vi "test Deployment Import Configuration.vi"(8 "error in":errorcluster, 11 "TestCase in":refnum<class "Deployment.lvclass">) -> (0 "error out":errorcluster, 3 "TestCase out":refnum<class "Deployment.lvclass">)   [LabVIEW 2020, in "Deployment.lvclass"]
uses:
  Deployment.lvclass
  <vilib>/addons/_JKI Toolkits/VI Tester/TestCase.llb/TestCase.lvclass
  315b1c3a-44c8-49e8-b756-01f865c29b4a.vi
  niveristand-custom-device-testing-tools/VeriStandTestUtilities/VeriStandTestUtilities.lvlib
  Scripting/AIM MIL-STD-1553 Scripting.lvlib
  C:/Program Files (x86)/National Instruments/LabVIEW 2020/vi.lib/addons/_JKI Toolkits/VI Tester/TestCase.llb/TestCase.lvclass
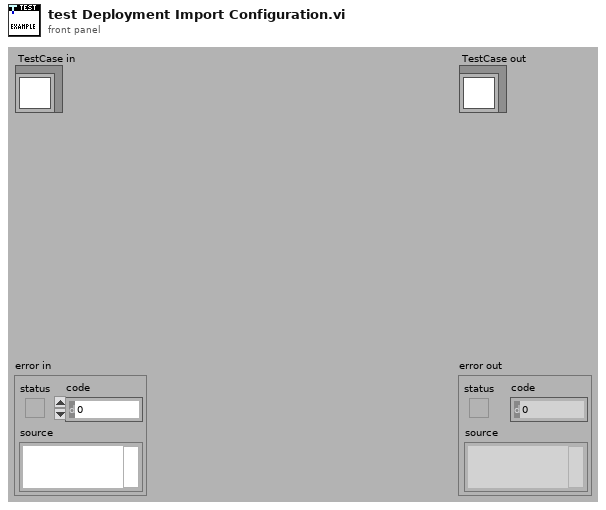
[diagram p1: front panel]
types:
  T1 = typedef "Custom Device API.lvlib/Custom Device Item Ref.ctl" = u64
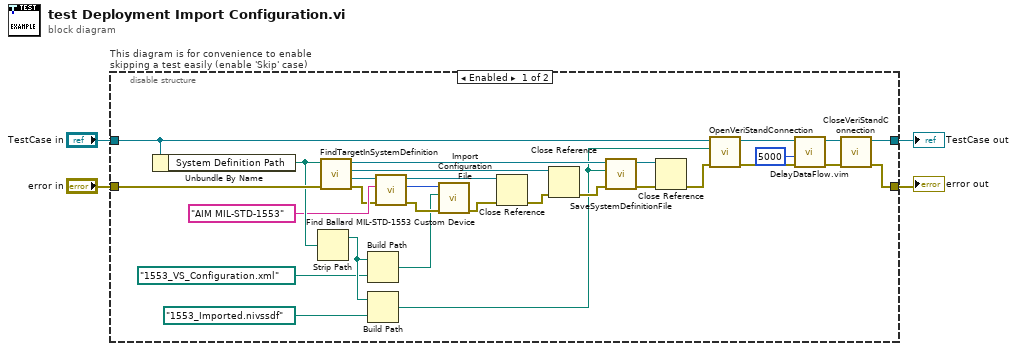
[diagram p0: block diagram]
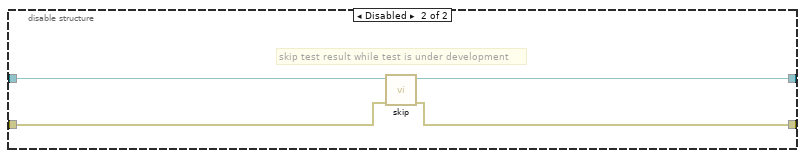
[diagram p2: hidden frame]
diagram:
  n1 = disable-structure "This diagram is for convenience to enable skipping a test easily (enable 'Skip' case)" shown="Enabled" {
    disable-tunnel: "TestCase in" -> [w26 w36]
    disable-tunnel: [w27 w34] -> w1
    disable-tunnel: [w29 w35] -> w3
    disable-tunnel: "error in" -> [w25 w33]
    frame Enabled {
      n2 = Unbundle By Name(w26) -> ("System Definition Path"=w23:path)
      n3 = Strip Path(path=w23) -> (stripped path=w8:path)  [unwired: 1 out]
      n4 = call "FindTargetInSystemDefinition.vi"("error in"=w25, "system definition path"=w23) -> ("error out"=w12:errorcluster, "Target"=w15:refnum<k24>, "Root"=w18:refnum<k24>, "System Definition"=w24:refnum<k24>)  [unwired: 6 in]
      n5 = Build Path(base path=w8, name or relative path=path "1553_VS_Configuration.xml") -> (appended path=w6:path)
      n6 = Build Path(base path=w8, name or relative path=path "1553_Imported.nivssdf") -> (appended path=w9:path)
      n7 = call "Find Ballard MIL-STD-1553 Custom Device.vi"("error in"=w12, "name"="AIM MIL-STD-1553", "target in"=w15) -> ("error out"=w10:errorcluster, "Ballard MIL-STD 1553 custom device"=w11:T1, "target out"=w13:refnum<k24>)  [unwired: 5 in, 1 out]
      n8 = call "Import Configuration File.vi"("error in"=w10, "parameters configuration file path"=w6, "custom device ref"=w11) -> ("error out"=w5:errorcluster)  [unwired: 7 in, 1 out]
      n9 = Close Reference(reference=w13, error in (no error)=w5) -> (error out=w16:errorcluster)
      n10 = Close Reference(reference=w18, error in (no error)=w16) -> (error out=w17:errorcluster)
      n11 = call "SaveSystemDefinitionFile.vi"("error in (no error)"=w17, "System Definition File in"=w9, "System Definition Reference in"=w24) -> ("error out"=w20:errorcluster, "System Definition Reference out"=w21:refnum<k24>)  [unwired: 7 in]
      n12 = Close Reference(reference=w21, error in (no error)=w20) -> (error out=w19:errorcluster)
      n13 = call-dynamic "OpenVeriStandConnection.vi"("error in (no error)"=w19, "System Definition File"=w9, "VeriStand Test Case in"=w26) -> ("error out"=w32:errorcluster, "VeriStand Test Case out"=w28:refnum<class "Deployment.lvclass">)  [unwired: 6 in, 1 out]
      n14 = call "DelayDataFlow.vim"("value in"=w32, "milliseconds to wait"=u32 5000) -> ("value out"=w30:errorcluster)  [unwired: 2 in, 1 out]
      n15 = call-dynamic "CloseVeriStandConnection.vi"("error in (no error)"=w30, "VeriStand Test Case in"=w28) -> ("error out"=w29:errorcluster, "VeriStand Test Case out"=w27:refnum<class "Deployment.lvclass">)  [unwired: 8 in]
    }
    frame Disabled {
      # "skip test result while test is under development"
      n16 = call <vilib>:"skip.vi"("error in (no error)"=w33, "TestCase in"=w36) -> ("error out"=w35:errorcluster, "TestCase out"=w34:refnum<class "Deployment.lvclass">)  [unwired: 8 in]
    }
  }
  "error out" <- w3
  "TestCase out" <- w1
